vi "10-send&receive-arrays.vi"() -> ()   [LabVIEW 2018, in "LV2Julia_examples.lvlib"]
uses:
  LV2Julia_examples.lvlib
  LV2Julia_core/VIs/Server or client state.ctl
  LV2Julia_core/VIs/detailed error info.ctl
  LV2Julia_core/VIs/StackFrame.ctl
  LV2Julia_core/VIs/Numeric Types enum.ctl
  array 123D sizes.ctl
  LV2Julia_core/VIs/Commands.ctl
  LV2Julia_core/VIs/ZMQ timeouts.ctl
  19565153-6e23-41a7-814d-e58de81dde5a.vi
  5ef99b4f-9bfc-4a0d-a8a0-74b261859f3d.vi
  388a3b2a-e541-4e37-ba3b-5749cefc77c1.vi
  e91abbe1-2489-4f0d-9743-379a6a4cbf4d.vi
  19565153-6e23-41a7-814d-e58de81dde5a.vi/85887d54-d509-450b-84bb-3c420582994f.vi
  <vilib>/Utility/High Resolution Relative Seconds.vi
  388a3b2a-e541-4e37-ba3b-5749cefc77c1.vi/1b30b06e-7fd1-4fdb-a624-ecc8bbac65c1.vi
  19565153-6e23-41a7-814d-e58de81dde5a.vi/85887d54-d509-450b-84bb-3c420582994f.vi/d3e8bd18-7aca-49eb-9cc1-8936944af3d1.vi
  19565153-6e23-41a7-814d-e58de81dde5a.vi/85887d54-d509-450b-84bb-3c420582994f.vi/cc0638ed-03b9-4f11-90bc-5f951413100e.vi
  19565153-6e23-41a7-814d-e58de81dde5a.vi/85887d54-d509-450b-84bb-3c420582994f.vi/437cd6de-f34e-42af-877a-dd33a1fabbe3.vi
  388a3b2a-e541-4e37-ba3b-5749cefc77c1.vi/1b30b06e-7fd1-4fdb-a624-ecc8bbac65c1.vi/cb39e787-6450-4332-a618-a02e848b2eda.vi
  388a3b2a-e541-4e37-ba3b-5749cefc77c1.vi/1b30b06e-7fd1-4fdb-a624-ecc8bbac65c1.vi/8ffec59d-6774-4d31-b6e2-7d50134dbb1f.vi
  388a3b2a-e541-4e37-ba3b-5749cefc77c1.vi/1b30b06e-7fd1-4fdb-a624-ecc8bbac65c1.vi/38fcd616-394b-4d55-b8d7-64853e38e30b.vi
  LV2Julia_core/VIs/jl-scripts path.vi
  LV2Julia_core/VIs/check ID validity.vi
  LV2Julia_core/VIs/bindata_descr to JSON.vi
  LV2Julia_core/VIs/check cluster field names.vi
  LV2Julia_core/VIs/concat JSON.vi
  LV2Julia_core/VIs/build request.vi
  LV2Julia_core/VIs/Parse server response.vi
  LV2Julia_core/VIs/log jl exceptions.vi
  LV2Julia_core/LV2Julia_core.lvlib
panel:
  out "ZMQ timeout":bool
  out "Julia script file path":path
  out "temporary script path":path
  in  "execution control pages":enum32{"Start&stop", "go - test", "error"}(tab)
  in  "go":bool caption="go (Julia Server started externally)"
  in  "Start with Julia":bool caption="Start Julia Server and go"
  in  "ZMQ endpoint":string="tcp://127.0.0.1:5555"
  out "Jl Server state":T1
  out "numarray 3D":cdb[][][](array[numeric])
  out "numarray 2D":cdb[][](array[numeric])
  out "numarray 1D":cdb[](array[numeric]) format="%.1f"
  out "numeric type":T2
  out "arr dimension":i32
  out "all arrays OK":bool
  out "arrs equal":bool
  out "array sizes":T3
  out "el_type":string
  out "arsize":i32[](array[numeric])
  out "data flattening delta t":dbl
  out "flattening ms/MB":dbl format="%#.2f"
  out "Zmq&Julia delta t":dbl
  out "Zmq&JUlia ms/MB":dbl format="%#.2f"
  out "data unflattening delta t":dbl
  out "unflattening ms/MB":dbl format="%#.2f"
  in  "stop VI":bool caption="stop this VI only"
  in  "stop both":bool caption="stop both this VI and Julia Server"
  in  "returnarrs":bool=TRUE
  in  "log2(arrsize)":u32=7 min=5
  in  "cycle min time (s)":sgl min=0 step=0.2
  in  "next":bool
  out "warm up":bool
  in  "test extent":enum32{"all types", "spec type"}(tab)
  in  "arr type":T2
  in  "dims":cluster{"1D":bool, "2D":bool, "3D":bool}
  in  "rounds":u32=1 min=1
  out "detailed error info":T4
  out "current error":errorcluster
  out "final error":errorcluster
  out "short err code":u8
  # "tcp://127.0.0.1:5555 \nfor local Julia Server\n\nFor a Julia Server running on a separate computer,  you probably must use an IPv4 address in numeric form (not a DNS name) - see https://stackoverflow.com/questions/6024003/why-doesnt-zeromq-work-on-localhost.\n\nFor instructions how to properly start the corresponding Julia script, see \n05-on_external_server.jl file in the jl-scripts folder.\n\nThe ZMQ endpoint control only used if Julia Server is not being started by this VI."
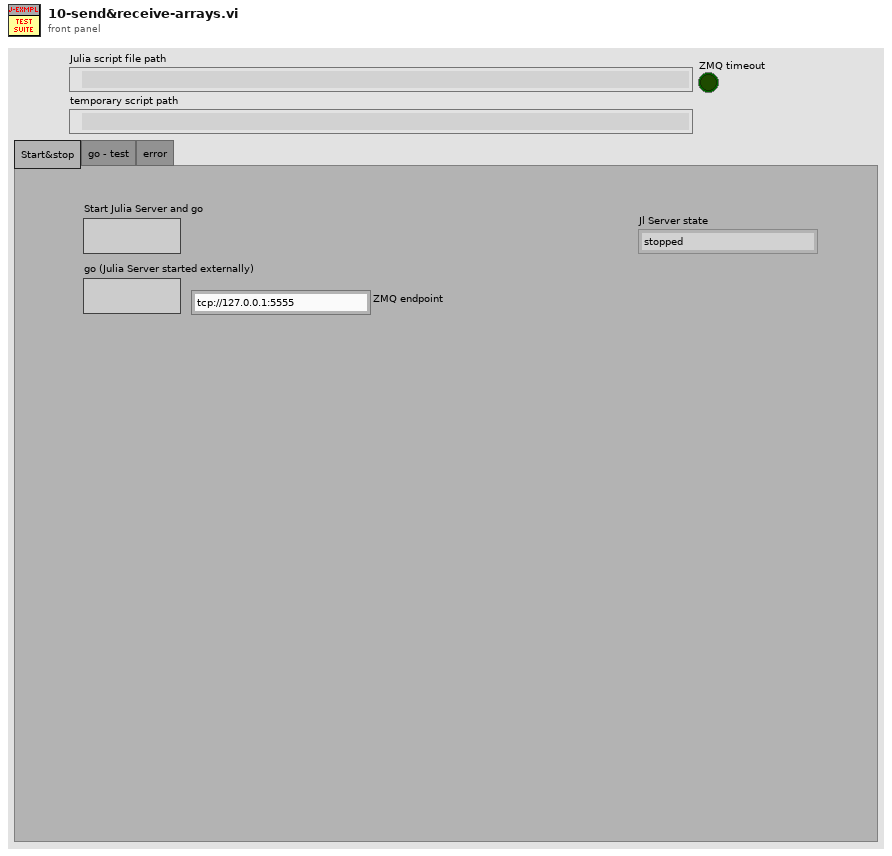
[diagram p1: front panel]
types:
  T1 = typedef "LV2Julia_core.lvlib/Server or client state.ctl" = enum16{"stopped", "running", "unknown"}
  T2 = typedef "LV2Julia_core.lvlib/Numeric Types enum.ctl" = enum16{"SGL", "DBL", "I8", "I16", "I32", "I64", "U8", "U16", "U32", "U64", "CSGL", "CDBL", "boolean"}
  T3 = typedef "LV2Julia_examples.lvlib/array 123D sizes.ctl" = cluster{"s1":i32, "s2":i32[], "s3":i32[]}
  T4 = typedef "LV2Julia_core.lvlib/detailed error info.ctl" = cluster{"exception_or_info":string, "trace":T5[]}
  T5 = typedef "LV2Julia_core.lvlib/StackFrame.ctl" = cluster{"frame_summary":string, "func":string, "linfo":string, "file":string, "line":i32, "pointer":u64, "from_c":bool, "inlined":bool}
  T6 = typedef "LV2Julia_core.lvlib/ZMQ timeouts.ctl" = cluster{"SNDTIMEO":i32, "RCVTIMEO":i32}
  T7 = typedef "LV2Julia_core.lvlib/Commands.ctl" = enum16{"Start Jl-server & Init LV-client", "Send request & Get response ", "Stop Jl-server & Cleanup LV-client", "Cleanup LV-client", "Start Jl-server", "Stop Jl-server", "Init LV-Client", "Cleanup LV-Client", "(not allowed)", "Set LV Client state", "Set Jl Server state", "set ZMQ timeout", "read ZMQ timeout", "read-out state"}
  T8 = typedef "LV2Julia_core.lvlib/Bindata&description.ctl" = cluster{"bindata_descr":T9[], "bindata":u8[]}
  T9 = typedef "LV2Julia_core.lvlib/Bindata description.ctl" = cluster{"nofbytes":i32, "numtype":string, "start":i32, "arrdims":i32[], "kwarg_name":string, "category":string}
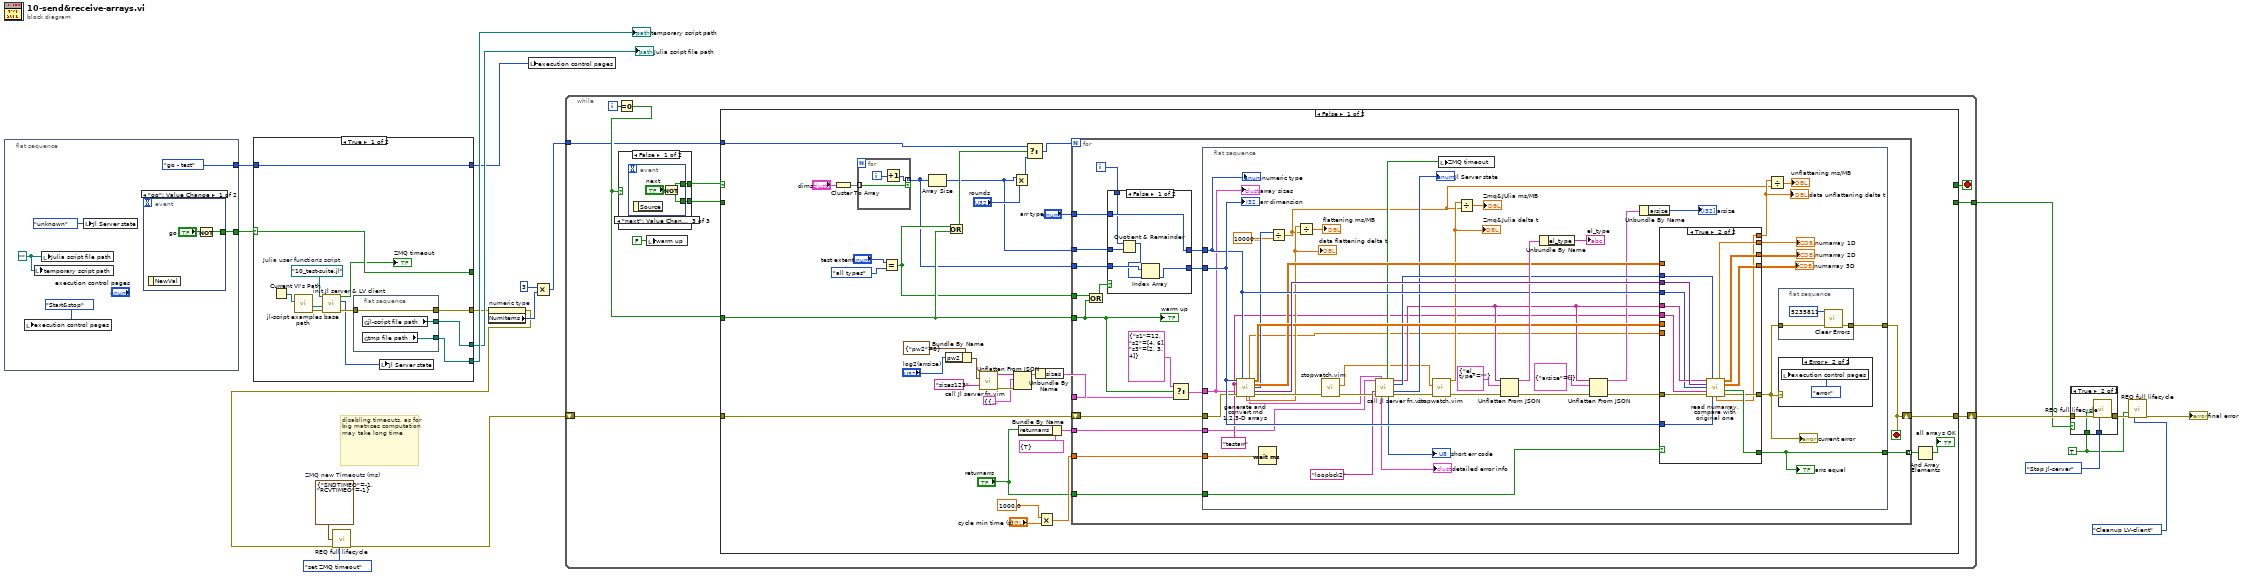
[diagram p0: block diagram]
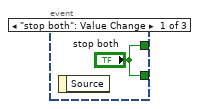
[diagram p2: hidden frame]
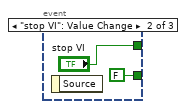
[diagram p3: hidden frame]
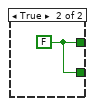
[diagram p4: hidden frame]
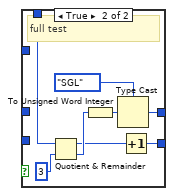
[diagram p5: hidden frame]
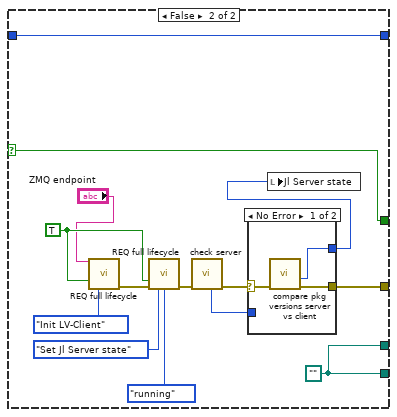
[diagram p9: hidden frame]
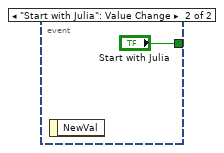
[diagram p11: hidden frame]
diagram:
  w3 = T6 {"SNDTIMEO"=-1, "RCVTIMEO"=-1}  # ZMQ new Timeouts (ms)
  w16 = TRUE ("Force command")
  # "disabling timeouts, as for big matrices computation may take long time"
  n1 = flat-sequence {
    tunnel: [w23] -> w12
    tunnel: [enum32{"Start&stop", "go - test", "error"}."go - test" ("execution control pages")] -> w7
    frame #0 {
      w24 = path ""
      n2 = local write "execution control pages"(enum32{"Start&stop", "go - test", "error"}."Start&stop" ("execution control pages")) -> ()
      n3 = local write "temporary script path"(w24) -> ()
      n4 = local write "Julia script file path"(w24) -> ()
      n5 = local write "Jl Server state"(Server_or_client_state."unknown" ("Jl Server state out")) -> ()
      n6 = event shown="[0] \"go\": Value Change" {
        selector: _ -> [_ _]
        dyn-events: _ -> [_ _]
        timeout: _ -> [_ _]
        tunnel: [w26 "Start with Julia"] -> w23
        event "go": Value Change {
          n7 = event-data() -> ()  [unwired: 1 in, 1 out]
          n8 = Not(x="go") -> (.not. x?=w26:bool)
        }
        event "Start with Julia": Value Change {
          n9 = event-data() -> ()  [unwired: 1 in, 1 out]
        }
      }
    }
  }
  n10 = case shown="True" w12 {
    selector: w12 -> [w40 w53]
    tunnel: [w39 w48] -> w9
    tunnel: [w40 w53] -> _
    tunnel: [w38 w50] -> w10
    tunnel: [w37 w50] -> w11
    tunnel: [w29 w44] -> w8
    tunnel: w7 -> [w29 w44]
    frame True {
      w31 = path "10_test-suite.jl"  # Julia user functions script
      n11 = Current VI's Path() -> (path=w35:path)
      n12 = call "jl-script examples base path.vi"("calling example VI path"=w35) -> ("error out"=w34:errorcluster, "jl-script-examples base path"=w33:path)  [unwired: 9 in]
      n13 = call "init Jl server & LV client.vi"("error in (no error)"=w34, "Base path (not a path)"=w33, "Julia user functions script"=w31) -> ("error out"=w36:errorcluster, "Jl Server state out"=w32:T1, "timeout?"=→"ZMQ timeout":bool)  [unwired: 6 in]
      n14 = flat-sequence {
        tunnel: [w43] -> w39
        tunnel: w36 -> [w43]
        tunnel: [w42] -> w38
        tunnel: [w41] -> w37
        frame #0 {
          n15 = global read "jl-scripts path.vi" "jl-script file path"() -> (w42:path)
          n16 = global read "jl-scripts path.vi" "tmp file path"() -> (w41:path)
        }
      }
      n17 = local write "Jl Server state"(w32) -> ()
    }
    frame False {
      w50 = path ""
      w55 = TRUE ("Force command")
      n18 = call "REQ full lifecycle.vi"("ZMQ endpoint"="ZMQ endpoint", "Force command"=w55, "command"=Commands."Init LV-Client") -> ("error out"=w52:errorcluster)  [unwired: 6 in, 6 out]
      n19 = call "REQ full lifecycle.vi"("Force command"=w55, "error in"=w52, "command"=Commands."Set Jl Server state", "Jl Server state in"=Server_or_client_state."running") -> ("error out"=w51:errorcluster)  [unwired: 5 in, 6 out]
      n20 = call "check server.vi"("error in"=w51) -> ("error out"=w49:errorcluster, "Jl Server state out"=w47:T1)  [unwired: 6 in, 3 out]
      n21 = case shown="No Error" w49 {
        selector: w49 -> [w60 w62]
        tunnel: [w59 w62] -> w48
        tunnel: [w58 w61] -> w45
        tunnel: w47 -> [_ w61]
        frame No Error {
          n22 = call "compare pkg versions server vs client.vi"("error in (no error)"=w60) -> ("error out"=w59:errorcluster, "Jl Server state out"=w58:T1)  [unwired: 4 in, 5 out]
        }
        frame Error {
        }
      }
      n23 = local write "Jl Server state"(w45) -> ()
    }
  }
  "temporary script path" <- w11
  "Julia script file path" <- w10
  n24 = property on="numeric type" class="Enum (strict)"(error in=w9) -> (error out=w1:errorcluster, "NumItems"=w15:u32)  [unwired: 1 in, 1 out]
  n25 = call "REQ full lifecycle.vi"("ZMQ new Timeouts in"=w3, "error in"=w1, "command"=Commands."set ZMQ timeout") -> ("error out"=w2:errorcluster)  [unwired: 6 in, 6 out]
  n26 = local write "execution control pages"(w8) -> ()
  n27 = Multiply(x=u32 3, y=w15) -> (x*y=w13:u32)
  n28 = while {
    tunnel: w13 -> [w63]
    shift-right: [w72] -> w6
    shift-left: w2 -> [w71]
    tunnel: [w69] -> w5
    i -> [w66]
    stop <- w67 stop-if-true
    n29 = Equal To 0?(x=w66) -> (x = 0?=w64:bool)
    n30 = case shown="False" w64 {
      tunnel: [w74 w80] -> w70
      tunnel: [w73 w80] -> w68
      frame False {
        n31 = event shown="[2] \"next\": Value Change" {
          selector: _ -> [_ _ _]
          dyn-events: _ -> [_ _ _]
          timeout: _ -> [_ _ _]
          tunnel: ["stop both" "stop VI" w78] -> w73
          tunnel: ["stop both" FALSE ("stop both this VI and Julia Server") w78] -> w74
          event "stop both": Value Change {
            n32 = event-data() -> ()  [unwired: 1 in, 1 out]
          }
          event "stop VI": Value Change {
            n33 = event-data() -> ()  [unwired: 1 in, 1 out]
          }
          event "next": Value Change {
            n34 = event-data() -> ()  [unwired: 1 in, 1 out]
            n35 = Not(x="next") -> (.not. x?=w78:bool)
          }
        }
      }
      frame True {
        w80 = FALSE ("stop this VI only")
      }
    }
    n36 = local write "warm up"(FALSE ("warm up")) -> ()
    n37 = case shown="False" w68 {
      selector: w68 -> [_ w219]
      tunnel: [w113 w218] -> w72
      tunnel: w71 -> [w112 w218]
      tunnel: [_ w220] -> w69
      tunnel: w70 -> [_ w220]
      tunnel: [_ w219] -> w67
      tunnel: w64 -> [w105 _]
      tunnel: w63 -> [w107 _]
      frame False {
        n38 = Cluster To Array(cluster="dims") -> (array=w86:bool[])
        n39 = for {
          tunnel: w86 -> [w114] mode=indexing
          tunnel: [w115] -> w81 mode=indexing if=w114
          i -> [w116]
          n40 = Increment(x=w116) -> (x+1=w115:i32)
        }
        n41 = Equal?(x="test extent", y=enum32{"all types", "spec type"}."all types" ("test extent")) -> (x = y?=w84:bool)
        n42 = Array Size(array=w81) -> (size(s)=w82:i32)
        n43 = Bundle By Name(cluster=cluster{"pw2":u32} {"pw2"=8}, "pw2"="log2(arrsize)") -> (w100:cluster{"pw2":u32})
        n44 = Or(x=w84, y=w105) -> (x .or. y?=w85:bool)
        n45 = call "call Jl server fn.vim"("Arguments 2"=w100, "fun2call"="sizes123") -> ("JSON received"=w103:string, "error out"=w104:errorcluster)  [unwired: 7 in, 5 out]
        n46 = Multiply(x=w82, y="rounds") -> (x*y=w83:u32)
        n47 = Unflatten From JSON(JSON string=w103, type and defaults=cluster{"sizes":T3} {"sizes"={"s1"=0, "s2"=[], "s3"=[]}}, error in (no error)=w104) -> (value=w102:cluster{"sizes":T3})  [unwired: 4 in, 1 out]
        n48 = Bundle By Name(cluster=cluster{"returnarrs":bool} {"returnarrs"=TRUE}, "returnarrs"="returnarrs") -> (w92:cluster{"returnarrs":bool})
        n49 = Select(t=w107, s=w85, f=w83) -> (s? t:f=w106:u32)
        n50 = Unbundle By Name(w102) -> ("sizes"=w96:T3)
        n51 = Multiply(x=sgl 1000.0, y="cycle min time (s)") -> (x*y=w93:sgl)
        n52 = for {
          N: w106 -> [_]
          tunnel: [w127] -> w111 mode=indexing
          shift-right: [w132] -> w113
          shift-left: w112 -> [w133]
          tunnel: w92 -> [w129]
          tunnel: "returnarrs" -> [w130]
          tunnel: w96 -> [w124]
          tunnel: w93 -> [w128]
          tunnel: w105 -> [w122]
          tunnel: "arr type" -> [w121]
          tunnel: w84 -> [w119]
          tunnel: w82 -> [w118]
          tunnel: w81 -> [w117]
          i -> [w126]
          stop <- w132 stop-if-true
          n53 = Or(x=w119, y=w122) -> (x .or. y?=w120:bool)
          n54 = case shown="False" w120 {
            tunnel: [w135 w143] -> w134
            tunnel: [w140 w142] -> w131
            tunnel: w126 -> [w138 w141]
            tunnel: w121 -> [w140 _]
            tunnel: w118 -> [w139 _]
            tunnel: w117 -> [w137 _]
            frame False {
              n55 = Quotient & Remainder(x=w138, y=w139) -> (x-y*floor(x/y)=w136:i32)  [unwired: 1 out]
              n56 = Index Array(array=w137, index=w136) -> (element=w135:i32)
            }
            frame True {
              # "full test"
              n57 = Quotient & Remainder(x=w141, y=3) -> (x-y*floor(x/y)=w144:i32, floor(x/y)=w145:i32)
              n58 = To Unsigned Word Integer(number=w145) -> (unsigned 16bit integer=w146:u16)
              n59 = Type Cast(type=Numeric_Types_enum."SGL" ("numeric type const"), x=w146) -> (*(type *) &x=w142:T2)
              n60 = Increment(x=w144) -> (x+1=w143:i32)
            }
          }
          n61 = Select(t=T3 {"s1"=12, "s2"=[4, 6], "s3"=[2, 3, 4]} ("f"), s=w122, f=w124) -> (s? t:f=w125:T3)
          n62 = flat-sequence {
            tunnel: w134 -> [w194]
            tunnel: w133 -> [w193]
            tunnel: [w192] -> w132
            tunnel: w131 -> [w188]
            tunnel: w130 -> [w185]
            tunnel: w129 -> [w152]
            tunnel: w125 -> [w153]
            tunnel: w128 -> [w176]
            tunnel: [w157] -> w127
            frame #0 {
              w154 = "testarr" ("Tag")
              n63 = call "generate and convert rnd 1,2,3-D arrays.vi"("dims"=w194, "numeric type const"=w188, "Tag"=w154, "sizes"=w153, "error in (no error)"=w193) -> ("Array 1D"=w149:cdb[], "Array 2D"=w184:cdb[][], "Array 3D"=w183:cdb[][][], "bytes"=w158:i32, "array as variant"=w196:variant, "delta t (s)"=w164:dbl, "Bindata & descr out"=w151:T8, "error out"=w168:errorcluster)  [unwired: 1 in, 2 out]
              "data flattening delta t" <- w164
              n64 = Wait (ms)(milliseconds to wait=w176) -> ()  [unwired: 1 out]
              n65 = Divide(x=w158, y=1000000000.0) -> (x/y=w155:dbl)
              n66 = Divide(x=w164, y=w155) -> (x/y=→"flattening ms/MB":dbl)
              n67 = call "stopwatch.vim"("anything in"=w168) -> ("copy of anything out"=w167:errorcluster, "current timepoint"=w169:dbl)  [unwired: 8 in, 1 out]
              n68 = call "call Jl server fn.vim"("Arguments 1"=w152, "Bindata & descr in"=w151, "fun2call"="loopbck2", "error in (no error)"=w167) -> ("timeout?"=w177:bool, "JSON received"=w173:string, "binary data received"=w180:u8[], "Jl Server state out"=→"Jl Server state":T1, "detailed error info"=→"detailed error info":T4, "return code"=→"short err code":u8, "error out"=w166:errorcluster)  [unwired: 5 in]
              n69 = call "stopwatch.vim"("anything in"=w166, "prev timepoint (0)"=w169) -> ("copy of anything out"=w165:errorcluster, "delta t (s)"=w161:dbl)  [unwired: 7 in, 1 out]
              "Zmq&Julia delta t" <- w161
              n70 = local write "ZMQ timeout"(w177) -> ()
              n71 = Divide(x=w161, y=w155) -> (x/y=→"Zmq&JUlia ms/MB":dbl)
              n72 = Unflatten From JSON(JSON string=w173, type and defaults=cluster{"el_type":string} {"el_type"=""} ("parsed response"), error in (no error)=w165) -> (value=w191:cluster{"el_type":string}, error out=w175:errorcluster)  [unwired: 4 in]
              n73 = Unbundle By Name(w191) -> ("el_type"=→"el_type":string)
              n74 = Unflatten From JSON(JSON string=w173, type and defaults=cluster{"arsize":i32[]} {"arsize"=[]} ("parsed response"), error in (no error)=w175) -> (value=w171:cluster{"arsize":i32[]}, error out=w174:errorcluster)  [unwired: 4 in]
              n75 = Unbundle By Name(w171) -> ("arsize"=→"arsize":i32[])
              n76 = case shown="True" w185 {
                tunnel: w180 -> [_ w213]
                tunnel: [w199 w212] -> w150
                tunnel: w196 -> [_ w211]
                tunnel: [w197 w210] -> w195
                tunnel: [_ w209] -> w157
                tunnel: w194 -> [_ w208]
                tunnel: w174 -> [w200 w207]
                tunnel: w173 -> [_ w206]
                tunnel: w154 -> [_ w205]
                tunnel: w188 -> [_ w204]
                tunnel: [w198 w203] -> w187
                tunnel: [w200 w202] -> w186
                tunnel: w149 -> [w199 _]
                tunnel: w184 -> [w198 _]
                tunnel: w183 -> [w197 _]
                tunnel: [_ w201] -> w159
                frame False {
                }
                frame True {
                  n77 = call "read numarray, compare with original one.vi"("JSON in"=w206, "binary data in"=w213, "array as variant in"=w211, "numeric type"=w204, "kwarg_name"=w205, "error in (no error)"=w207, "dims"=w208) -> ("numarray 1D"=w212:cdb[], "numarray 2D"=w203:cdb[][], "numarray 3D"=w210:cdb[][][], "arrays are equal"=w209:bool, "delta t (s)"=w201:dbl, "error out"=w202:errorcluster)  [unwired: 1 in, 2 out]
                }
              }
              "numarray 1D" <- w150
              "arrs equal" <- w157
              "numarray 2D" <- w187
              "numarray 3D" <- w195
              "current error" <- w186
              "data unflattening delta t" <- w159
              n78 = Divide(x=w159, y=w155) -> (x/y=→"unflattening ms/MB":dbl)
              n79 = flat-sequence {
                tunnel: w186 -> [w217]
                tunnel: [w216] -> w192
                frame #0 {
                  n80 = call <vilib>:"Clear Errors.vi"("error in (no error)"=w217, "specific error code to clear (0: all)"=5235811) -> ("error out"=w216:errorcluster)  [unwired: 4 in, 1 out]
                }
              }
              n81 = case shown="Error" w186 {
                frame No Error {
                }
                frame Error {
                  n82 = local write "execution control pages"(enum32{"Start&stop", "go - test", "error"}."error" ("execution control pages")) -> ()
                }
              }
              "numeric type" <- w188
              "arr dimension" <- w194
              "array sizes" <- w153
            }
          }
          "warm up" <- w122
        }
        n83 = And Array Elements(Boolean array=w111) -> (logical AND=→"all arrays OK":bool)
      }
      frame True {
        # "stop"
      }
    }
  }
  n84 = case shown="True" w5 {
    tunnel: w6 -> [w221 w225]
    tunnel: Commands."Stop Jl-server" ("command") -> [_ w224]
    tunnel: [w221 w223] -> w19
    tunnel: w16 -> [_ w222]
    frame False {
    }
    frame True {
      n85 = call "REQ full lifecycle.vi"("Force command"=w222, "error in"=w225, "command"=w224) -> ("error out"=w223:errorcluster)  [unwired: 6 in, 6 out]
    }
  }
  n86 = call "REQ full lifecycle.vi"("Force command"=w16, "error in"=w19, "command"=Commands."Cleanup LV-client") -> ("error out"=→"final error":errorcluster)  [unwired: 6 in, 6 out]
